vi "Parse TCP-IP Response 4.vi"(0 "TCP/IP ID":refnum<k5>, 7 "timeout ms (5000)":i32=5000, 11 "error in (no error)":errorcluster) -> (1 "Header":string, 2 "Packet Error Code":i32, 3 "Packet ID":u8, 4 "Data Type":u16, 6 "Command Done":cluster{"Function #":u16}, 8 "Acq. Status":T3, 10 "Image Packet":T2, 12 "Status Array":sgl[](array[numeric]), 13 "Camera ID":u8, 14 "SI Image Settings":T1, 15 "error out":errorcluster)   [LabVIEW 2015]
uses:
  TCP-IP Image Packet.ctl
  SI Image Settings 1.ctl
panel:
  out "TCP/IP String":string
  out "Packet Length":u32
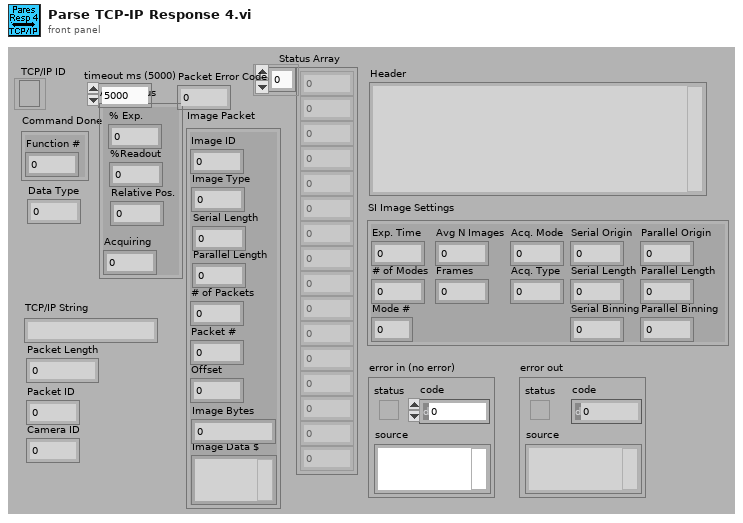
[diagram p1: front panel]
types:
  T1 = typedef "SI Image Settings 1.ctl" = cluster{"Exp. Time":u32, "# of Modes":u8, "Mode #":u8, "Avg N Images":u32, "Frames":u32, "Acq. Mode":u16, "Acq. Type":u16, "Serial Origin":i32, "Serial Length":i32, "Serial Binning":i32, "Parallel Origin":i32, "Parallel Length":i32, "Parallel Binning":i32}
  T2 = typedef "TCP-IP Image Packet.ctl" = cluster{"Image ID":u16, "Image Type":u16, "Serial Length":u16, "Parallel Length":u16, "# of Packets":u16, "Packet #":u16, "Offset":u32, "Image Bytes":u32, "Image Data $":string}
  T3 = cluster{"% Exp.":u16, "%Readout":u16, "Relative Pos.":u32, "Acquiring":dbl}
  T4 = enum16{"Standard", "Buffered", "CRLF", "Immediate"}
  T5 = cluster{"Image ID":u16, "Image Type":u16, "Serial Length":u16, "Parallel Length":u16, "# of Packets":u16, "Packet #":u16, "Offset":u32, "Image Bytes":u32}
  T6 = cluster{"Image ID":u16, "Image Type":u16, "Serial Length":u16, "Parallel Length":u16, "# of Packets":u16, "Packet #":u16, "Offset":u32, "Image Bytes":u32, "data out":string}
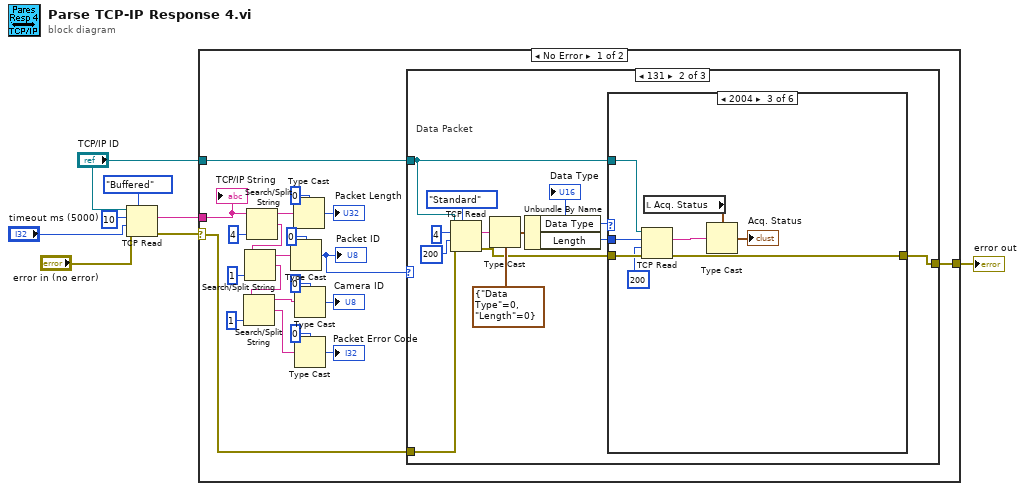
[diagram p0: block diagram]
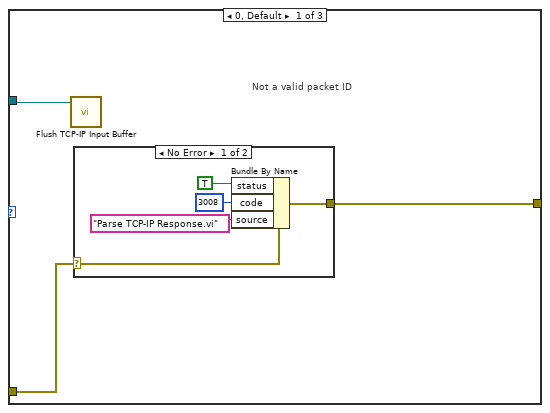
[diagram p2: hidden frame]
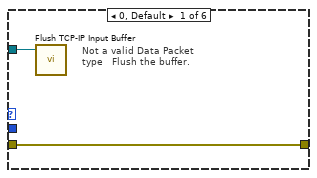
[diagram p4: hidden frame]
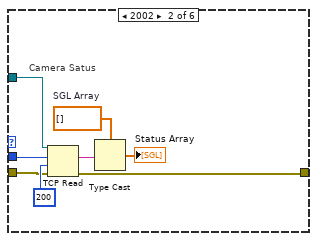
[diagram p5: hidden frame]
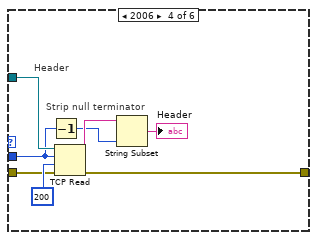
[diagram p6: hidden frame]
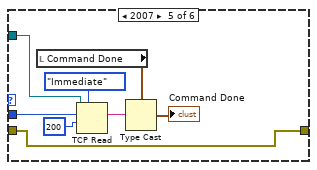
[diagram p7: hidden frame]
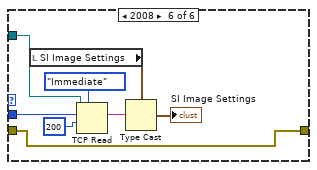
[diagram p8: hidden frame]
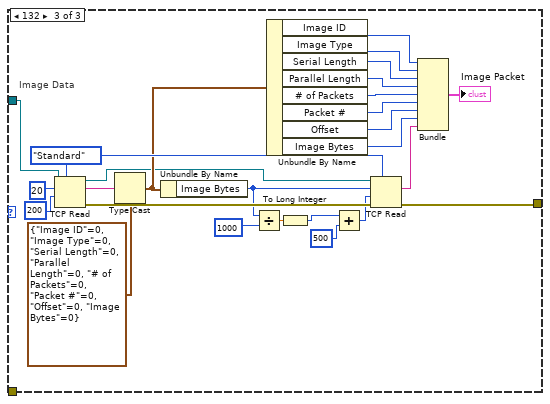
[diagram p9: hidden frame]
diagram:
  n1 = TCP Read(connection ID="TCP/IP ID", bytes to read=10, error in (no error)="error in (no error)", 7:T4."Buffered" ("mode (standard)"), 9:"timeout ms (5000)") -> (data out=w6:string, error out=w2:errorcluster)  [unwired: 1 out]
  n2 = case shown="No Error" w2 {
    selector: w2 -> [w15 w119]
    tunnel: w6 -> [w19 _]
    tunnel: "TCP/IP ID" -> [w17 _]
    tunnel: [w16 w119] -> w4
    frame No Error {
      n3 = Search/Split String(string=w19, offset (0)=4) -> (substring before match=w23:string, match + rest of string=w22:string)  [unwired: 1 in, 1 out]
      n4 = Search/Split String(string=w22, offset (0)=u16 1 ("default (0L)")) -> (substring before match=w24:string, match + rest of string=w13:string)  [unwired: 1 in, 1 out]
      n5 = Search/Split String(string=w13, offset (0)=u16 1 ("default (0L)")) -> (substring before match=w12:string, match + rest of string=w10:string)  [unwired: 1 in, 1 out]
      n6 = Type Cast(type=u8 0 ("default (0L)"), x=w24) -> (*(type *) &x=w18:u8)
      "Packet ID" <- w18
      n7 = Type Cast(type=u32 0 ("default (0L)"), x=w23) -> (*(type *) &x=→"Packet Length":u32)
      n8 = Type Cast(type=u8 0 ("default (0L)"), x=w12) -> (*(type *) &x=→"Camera ID":u8)
      n9 = Type Cast(type=0 ("default (0L)"), x=w10) -> (*(type *) &x=→"Packet Error Code":i32)
      n10 = case shown="131" w18 {
        tunnel: w17 -> [w30 w42 w101]
        tunnel: w15 -> [w31 w47 _]
        tunnel: [w32 w39 w113] -> w16
        frame 0, Default {
          # "Not a valid packet ID"
          n11 = call "Flush TCP-IP Input Buffer.vi"("TCP/IP ID"=w30) -> ()  [unwired: 4 in, 1 out]
          n12 = case shown="No Error" w31 {
            selector: w31 -> [w33 w38]
            tunnel: [w37 w38] -> w32
            frame No Error {
              n13 = Bundle By Name(cluster=w33, "status"=TRUE, "code"=3008, "source"="Parse TCP-IP Response.vi") -> (w37:errorcluster)
            }
            frame Error {
            }
          }
        }
        frame 131 {
          # "Data Packet"
          n14 = TCP Read(connection ID=w42, bytes to read=4, error in (no error)=w47, 7:T4."Standard" ("mode (standard)"), 9:200 ("timeout ms (25000)")) -> (data out=w46:string, error out=w40:errorcluster)  [unwired: 1 out]
          n15 = Type Cast(type=cluster{"Data Type":u16, "Length":u16} {"Data Type"=0, "Length"=0}, x=w46) -> (*(type *) &x=w44:cluster{"Data Type":u16, "Length":u16})
          n16 = Unbundle By Name(w44) -> ("Data Type"=w43:u16, "Length"=w41:u16)
          "Data Type" <- w43
          n17 = case shown="2004" w43 {
            tunnel: w42 -> [w51 w57 w68 w73 w79 w88]
            tunnel: w41 -> [_ w58 w67 w71 w78 w87]
            tunnel: w40 -> [w52 w59 w66 w75 w77 w86]
            tunnel: [w52 w56 w64 w74 w77 w86] -> w39
            frame 0, Default {
              # "Not a valid Data Packet type   Flush the buffer."
              n18 = call "Flush TCP-IP Input Buffer.vi"("TCP/IP ID"=w51) -> ()  [unwired: 4 in, 1 out]
            }
            frame 2002 {
              w54 = sgl[] []  # SGL Array
              # "Camera Satus"
              n19 = TCP Read(connection ID=w57, bytes to read=w58, error in (no error)=w59, 9:200 ("timeout ms (25000)")) -> (data out=w55:string, error out=w56:errorcluster)  [unwired: 1 in, 1 out]
              n20 = Type Cast(type=w54, x=w55) -> (*(type *) &x=→"Status Array":sgl[])
            }
            frame 2004 {
              n21 = TCP Read(connection ID=w68, bytes to read=w67, error in (no error)=w66, 9:200 ("timeout ms (25000)")) -> (data out=w65:string, error out=w64:errorcluster)  [unwired: 1 in, 1 out]
              n22 = local read "Acq. Status"() -> (w61:T3)
              n23 = Type Cast(type=w61, x=w65) -> (*(type *) &x=→"Acq. Status":T3)
            }
            frame 2006 {
              # "Strip null terminator"
              # "Header"
              n24 = Decrement(x=w71) -> (x-1=w70:u16)
              n25 = TCP Read(connection ID=w73, bytes to read=w71, error in (no error)=w75, 9:200 ("timeout ms (25000)")) -> (data out=w72:string, error out=w74:errorcluster)  [unwired: 1 in, 1 out]
              n26 = String Subset(string=w72, length (rest)=w70) -> (substring=→"Header":string)  [unwired: 1 in]
            }
            frame 2007 {
              n27 = local read "Command Done"() -> (w81:cluster{"Function #":u16})
              n28 = TCP Read(connection ID=w79, bytes to read=w78, 7:T4."Immediate" ("mode (standard)"), 9:200 ("timeout ms (25000)")) -> (data out=w82:string)  [unwired: 1 in, 2 out]
              n29 = Type Cast(type=w81, x=w82) -> (*(type *) &x=→"Command Done":cluster{"Function #":u16})
            }
            frame 2008 {
              n30 = local read "SI Image Settings"() -> (w89:T1)
              n31 = TCP Read(connection ID=w88, bytes to read=w87, 7:T4."Immediate" ("mode (standard)"), 9:200 ("timeout ms (25000)")) -> (data out=w90:string)  [unwired: 1 in, 2 out]
              n32 = Type Cast(type=w89, x=w90) -> (*(type *) &x=→"SI Image Settings":T1)
            }
          }
        }
        frame 132 {
          w117 = T4."Standard" ("mode (standard)")
          # "Image Data"
          n33 = TCP Read(connection ID=w101, bytes to read=20, 7:w117, 9:200 ("timeout ms (25000)")) -> (connection ID out=w102:refnum<k5>, data out=w115:string, error out=w114:errorcluster)  [unwired: 1 in]
          n34 = Type Cast(type=T5 {"Image ID"=0, "Image Type"=0, "Serial Length"=0, "Parallel Length"=0, "# of Packets"=0, "Packet #"=0, "Offset"=0, "Image Bytes"=0} ("*(type *) &x"), x=w115) -> (*(type *) &x=w103:T5)
          n35 = Unbundle By Name(w103) -> ("Image Bytes"=w100:u32)
          n36 = Divide(x=w100, y=1000 ("timeout ms (25000)")) -> (x/y=w98:dbl)
          n37 = Unbundle By Name(w103) -> ("Image ID"=w111:u16, "Image Type"=w110:u16, "Serial Length"=w109:u16, "Parallel Length"=w108:u16, "# of Packets"=w107:u16, "Packet #"=w106:u16, "Offset"=w96:u32, "Image Bytes"=w95:u32)
          n38 = To Long Integer(number=w98) -> (32bit integer=w97:i32)
          n39 = Add(x=w97, y=500) -> (x+y=w94:i32)
          n40 = TCP Read(connection ID=w102, bytes to read=w100, error in (no error)=w114, 7:w117, 9:w94) -> (data out=w105:string, error out=w113:errorcluster)  [unwired: 1 out]
          n41 = Bundle("Image ID"=w111, "Image Type"=w110, "Serial Length"=w109, "Parallel Length"=w108, "# of Packets"=w107, "Packet #"=w106, "Offset"=w96, "Image Bytes"=w95, "data out"=w105) -> (→"Image Packet":T6)  [unwired: 1 in]
        }
      }
      "TCP/IP String" <- w19
    }
    frame Error {
    }
  }
  "error out" <- w4
